vi "K2400_Output.vi"(2 "error in":errorcluster, 3 "Vg_Output":bool=TRUE, 4 "address (24)":string="24") -> (0 "error out":errorcluster)   [LabVIEW 2021]
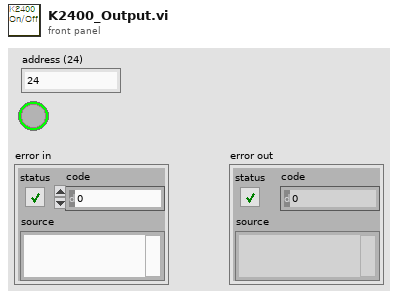
[diagram p1: front panel]
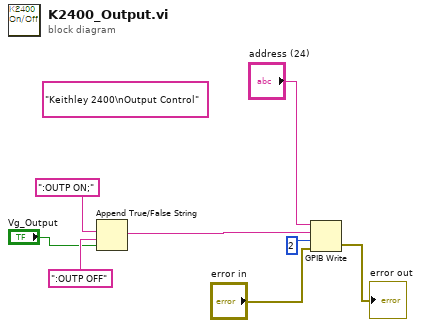
[diagram p0: block diagram]
diagram:
  (unwired) "Keithley 2400\nOutput Control"
  n1 = Append True/False String(1:"Vg_Output", 2:":OUTP OFF", 3:":OUTP ON;") -> (0:w8:string)  [unwired: 1 in]
  n2 = GPIB Write(0:"address (24)", 1:w8, 2:2, 3:"error in") -> (6:→"error out":errorcluster)  [unwired: 1 in, 1 out]
